vi "TCP_ReceiveFromGUI.vi"() -> ()   [LabVIEW 2018]
panel:
  in  "stop 2":bool
  out "error out":errorcluster
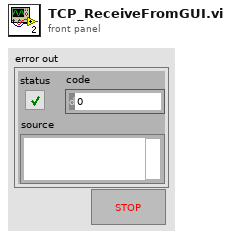
[diagram p1: front panel]
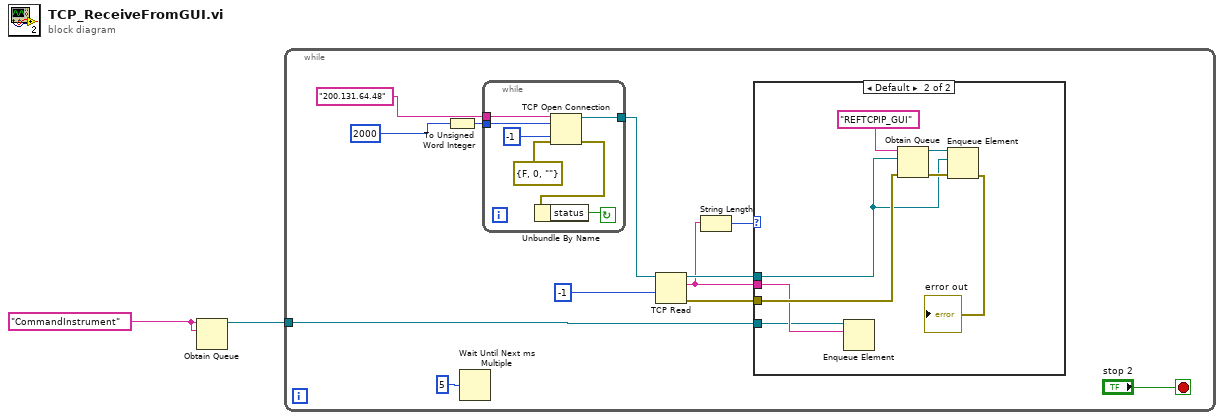
[diagram p0: block diagram]
diagram:
  w1 = "CommandInstrument"
  n1 = Obtain Queue(name (unnamed)=w1, element data type=w1) -> (queue out=w2:refnum<queue>)  [unwired: 3 in, 2 out]
  n2 = while {
    tunnel: w2 -> [w5]
    stop <- "stop 2" stop-if-true
    n3 = To Unsigned Word Integer(number=u32 2000 ("Remote Port:")) -> (unsigned 16bit integer=w8:u16)
    n4 = Wait Until Next ms Multiple(millisecond multiple=u32 5) -> ()  [unwired: 1 out]
    n5 = while {
      tunnel: [w29] -> w12
      tunnel: w8 -> [w28]
      tunnel: "200.131.64.48" ("Address:") -> [w27]
      stop <- w23 continue-if-true
      n6 = TCP Open Connection(address=w27, remote port or service name=w28, timeout ms (60000)=-1, error in (no error)=errorcluster {"status"=FALSE, "code"=0, "source"=""}) -> (connection ID=w29:refnum<k5>, error out=w24:errorcluster)  [unwired: 1 in]
      n7 = Unbundle By Name(w24) -> ("status"=w23:bool)
    }
    n8 = TCP Read(connection ID=w12, 9:-1 ("timeout ms (25000)")) -> (connection ID out=w10:refnum<k5>, data out=w3:string, error out=w11:errorcluster)  [unwired: 3 in]
    n9 = String Length(string=w3) -> (length=w4:i32)
    n10 = case shown="Default" w4 {
      tunnel: w11 -> [_ w21]
      tunnel: w10 -> [_ w19]
      tunnel: w3 -> [_ w16]
      tunnel: w5 -> [_ w15]
      frame 0 {
      }
      frame Default {
        n11 = Enqueue Element(queue=w15, element=w16) -> ()  [unwired: 2 in, 3 out]
        n12 = Obtain Queue(name (unnamed)="REFTCPIP_GUI", element data type=w19, error in (no error)=w21) -> (queue out=w18:refnum<queue>, error out=w20:errorcluster)  [unwired: 2 in, 1 out]
        n13 = Enqueue Element(queue=w18, element=w19, error in (no error)=w20) -> (error out=→"error out":errorcluster)  [unwired: 1 in, 2 out]
      }
    }
  }
